vi "edit io channel.vi"(8 "error in":errorcluster, 9 "line":T1, 10 "engine configuration in":refnum<class "engine configuration.lvclass">, 11 "tag bus configurable plugin module configuration in":refnum<class "tag bus configurable plugin module configuration.lvclass">) -> (0 "error out":errorcluster, 1 "change?":bool, 2 "engine configuration":refnum<class "engine configuration.lvclass">, 3 "tag bus configurable plugin module configuration out":refnum<class "tag bus configurable plugin module configuration.lvclass">)   [LabVIEW 2013]
uses:
  tag bus configurable plugin editor node.lvclass
  module/configuration/tag bus configurable plugin module configuration.lvclass
  <vilib>/NI/Module Execution Interface/Engine Configuration/engine configuration.lvclass
  <vilib>/NI/Tag Bus/tag/tag descriptor.lvclass
  <vilib>/NI/Configuration Framework/serializable configuration/NISE_CEF_serializable configuration.lvclass
  <vilib>/NI/Tag Bus Module Framework/channel/TBM channel.lvclass
  Mappings.ctl
  module/configuration/Line.ctl
  Map.ctl
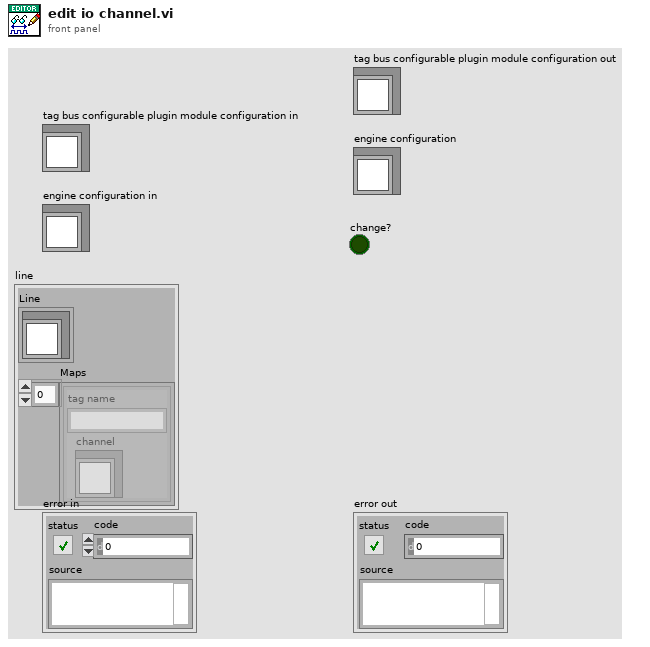
[diagram p1: front panel]
types:
  T1 = typedef "tag bus configurable plugin editor node.lvclass/Mappings.ctl" = cluster{"Line":T2, "Maps":T3[]}
  T2 = typedef "tag bus configurable plugin module configuration.lvclass/Line.ctl" = cluster{"channel":refnum<class "TBM channel.lvclass">}
  T3 = typedef "tag bus configurable plugin editor node.lvclass/Map.ctl" = cluster{"channel":refnum<class "TBM channel.lvclass">, "tag name":string}
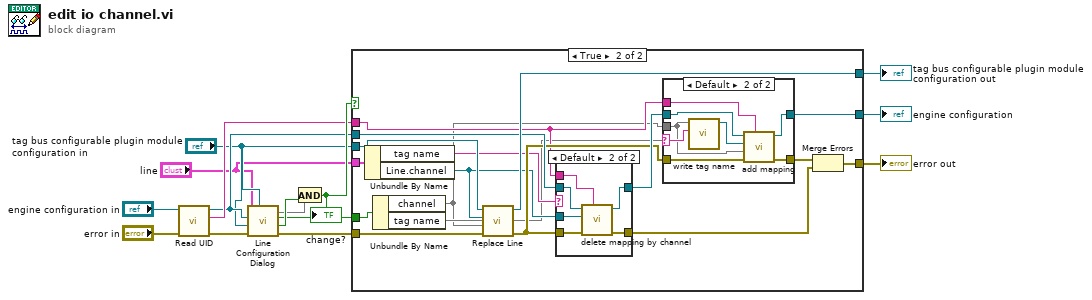
[diagram p0: block diagram]
diagram:
  n1 = call <vilib>:"Read UID.vi"("error in"="error in", "configuration in"="engine configuration in") -> ("error out"=w6:errorcluster, "instance id"=w4:string, "configuration out"=w3:refnum<class "engine configuration.lvclass">)  [unwired: 7 in]
  n2 = call "Line Configuration Dialog.vi"(7:"tag bus configurable plugin module configuration in", "error in"=w6, "engine configuration in"="tag bus configurable plugin module configuration in", "tag bus configurable plugin module configuration"=w3, "Line"="line") -> ("error out"=w9:errorcluster, "success"=w12:bool, "changed"=w10:bool, 5:w11)  [unwired: 2 in, 1 out]
  n3 = And(x=w11, y=w12) -> (x .and. y?=w13:bool)
  "change?" <- w13
  n4 = case shown="True" w13 {
    tunnel: [w17 w25] -> w7
    tunnel: [w18 w28] -> w15
    tunnel: w3 -> [w18 w30]
    tunnel: w9 -> [w17 w32]
    tunnel: w10 -> [_ w34]
    tunnel: "line" -> [_ w33]
    tunnel: "tag bus configurable plugin module configuration in" -> [w16 w35]
    tunnel: [w16 w31] -> w14
    tunnel: w4 -> [_ w21]
    frame False {
    }
    frame True {
      n5 = Unbundle By Name(w33) -> ("tag name"=w23:string, "Line.channel"=w22:refnum<class "TBM channel.lvclass">)
      n6 = Unbundle By Name(w34) -> ("channel"=w19, "tag name"=w20)
      n7 = call "Replace Line.vi"("error in"=w32, "New Line"=w19, "Line Name"=w22, "tag bus configurable plugin module configuration in"=w35) -> ("error out"=w24:errorcluster, "tag bus configurable plugin module configuration out"=w31:refnum<class "tag bus configurable plugin module configuration.lvclass">)  [unwired: 5 in, 1 out]
      n8 = case shown="Default" w23 {
        tunnel: w21 -> [_ w53]
        tunnel: w30 -> [w47 w52]
        tunnel: [w47 w51] -> w29
        tunnel: [w46 w50] -> w27
        tunnel: w24 -> [w46 w49]
        tunnel: w22 -> [_ w48]
        frame "" {
        }
        frame Default {
          n9 = call <vilib>:"delete mapping by channel.vi"("owner ID"=w53, "error in"=w49, "channel"=w48, "engine configuration in"=w52) -> ("error out"=w50:errorcluster, "engine configuration out"=w51:refnum<class "engine configuration.lvclass">)  [unwired: 6 in]
        }
      }
      n10 = case shown="Default" w20 {
        selector: w20 -> [_ w39]
        tunnel: w29 -> [w37 w45]
        tunnel: [w37 w44] -> w28
        tunnel: [w36 w43] -> w26
        tunnel: w24 -> [w36 w42]
        tunnel: w21 -> [_ w41]
        tunnel: w19 -> [_ w38]
        frame "" {
        }
        frame Default {
          n11 = call <vilib>:"write tag name.vi"("name"=w39, "system tag in"=w38) -> ("system tag out"=w40:refnum<class "tag descriptor.lvclass">)  [unwired: 8 in, 1 out]
          n12 = call <vilib>:"add mapping.vi"("owner ID"=w41, "error in"=w42, "channel"=w38, "tag descriptor"=w40, "engine configuration"=w45) -> ("error out"=w43:errorcluster, "engine configuration out"=w44:refnum<class "engine configuration.lvclass">)  [unwired: 5 in]
        }
      }
      n13 = Merge Errors(w26, w27) -> (w25:errorcluster)
    }
  }
  "engine configuration" <- w15
  "tag bus configurable plugin module configuration out" <- w14
  "error out" <- w7
